vi "Verify Matching Board Capabilities.vi"(0 "TX Board Settings":T1[](array[typedef]) {"Address Space" items=["VXI/VME A16"=1, "VXI/VME A24"=2, "VXI/VME A32"=3, "VXI/VME A64"=4, "PXI Memory Allocations"=9, "PXI Configuration"=10, "PXI BAR0"=11, "PXI BAR1"=12, "PXI BAR2"=13, "PXI BAR3"=14, "PXI BAR4"=15, "PXI BAR5"=16]}, 1 "RX Board Settings":T1[](array[typedef]) {"Address Space" items=["VXI/VME A16"=1, "VXI/VME A24"=2, "VXI/VME A32"=3, "VXI/VME A64"=4, "PXI Memory Allocations"=9, "PXI Configuration"=10, "PXI BAR0"=11, "PXI BAR1"=12, "PXI BAR2"=13, "PXI BAR3"=14, "PXI BAR4"=15, "PXI BAR5"=16]}, 11 "error in (no error)":errorcluster) -> (4 "RX TX Board Settings":T1[](array[typedef]) {"Address Space" items=["VXI/VME A16"=1, "VXI/VME A24"=2, "VXI/VME A32"=3, "VXI/VME A64"=4, "PXI Memory Allocations"=9, "PXI Configuration"=10, "PXI BAR0"=11, "PXI BAR1"=12, "PXI BAR2"=13, "PXI BAR3"=14, "PXI BAR4"=15, "PXI BAR5"=16]}, 15 "error out":errorcluster)   [LabVIEW 2019]
uses:
  <instrlib>/niMmWave/ni3610 and ni3630/controls/public/Main Settings.ctl
  <vilib>/Instr/_visa.llb/VISA Register Access Address Space.ctl
  <instrlib>/niMmWave/ni3610 and ni3630/controls/public/Register Adresses.ctl
  <instrlib>/niMmWave/ni3610 and ni3630/controls/public/Base Card Type.ctl
  <instrlib>/niMmWave/ni3610 and ni3630/controls/private/IQ Card Revision.ctl
  <instrlib>/niMmWave/ni3610 and ni3630/controls/public/Board Capability.ctl
  <instrlib>/niMmWave/ni3610 and ni3630/ni3610_and_ni3630_Driver_Lib.lvlib
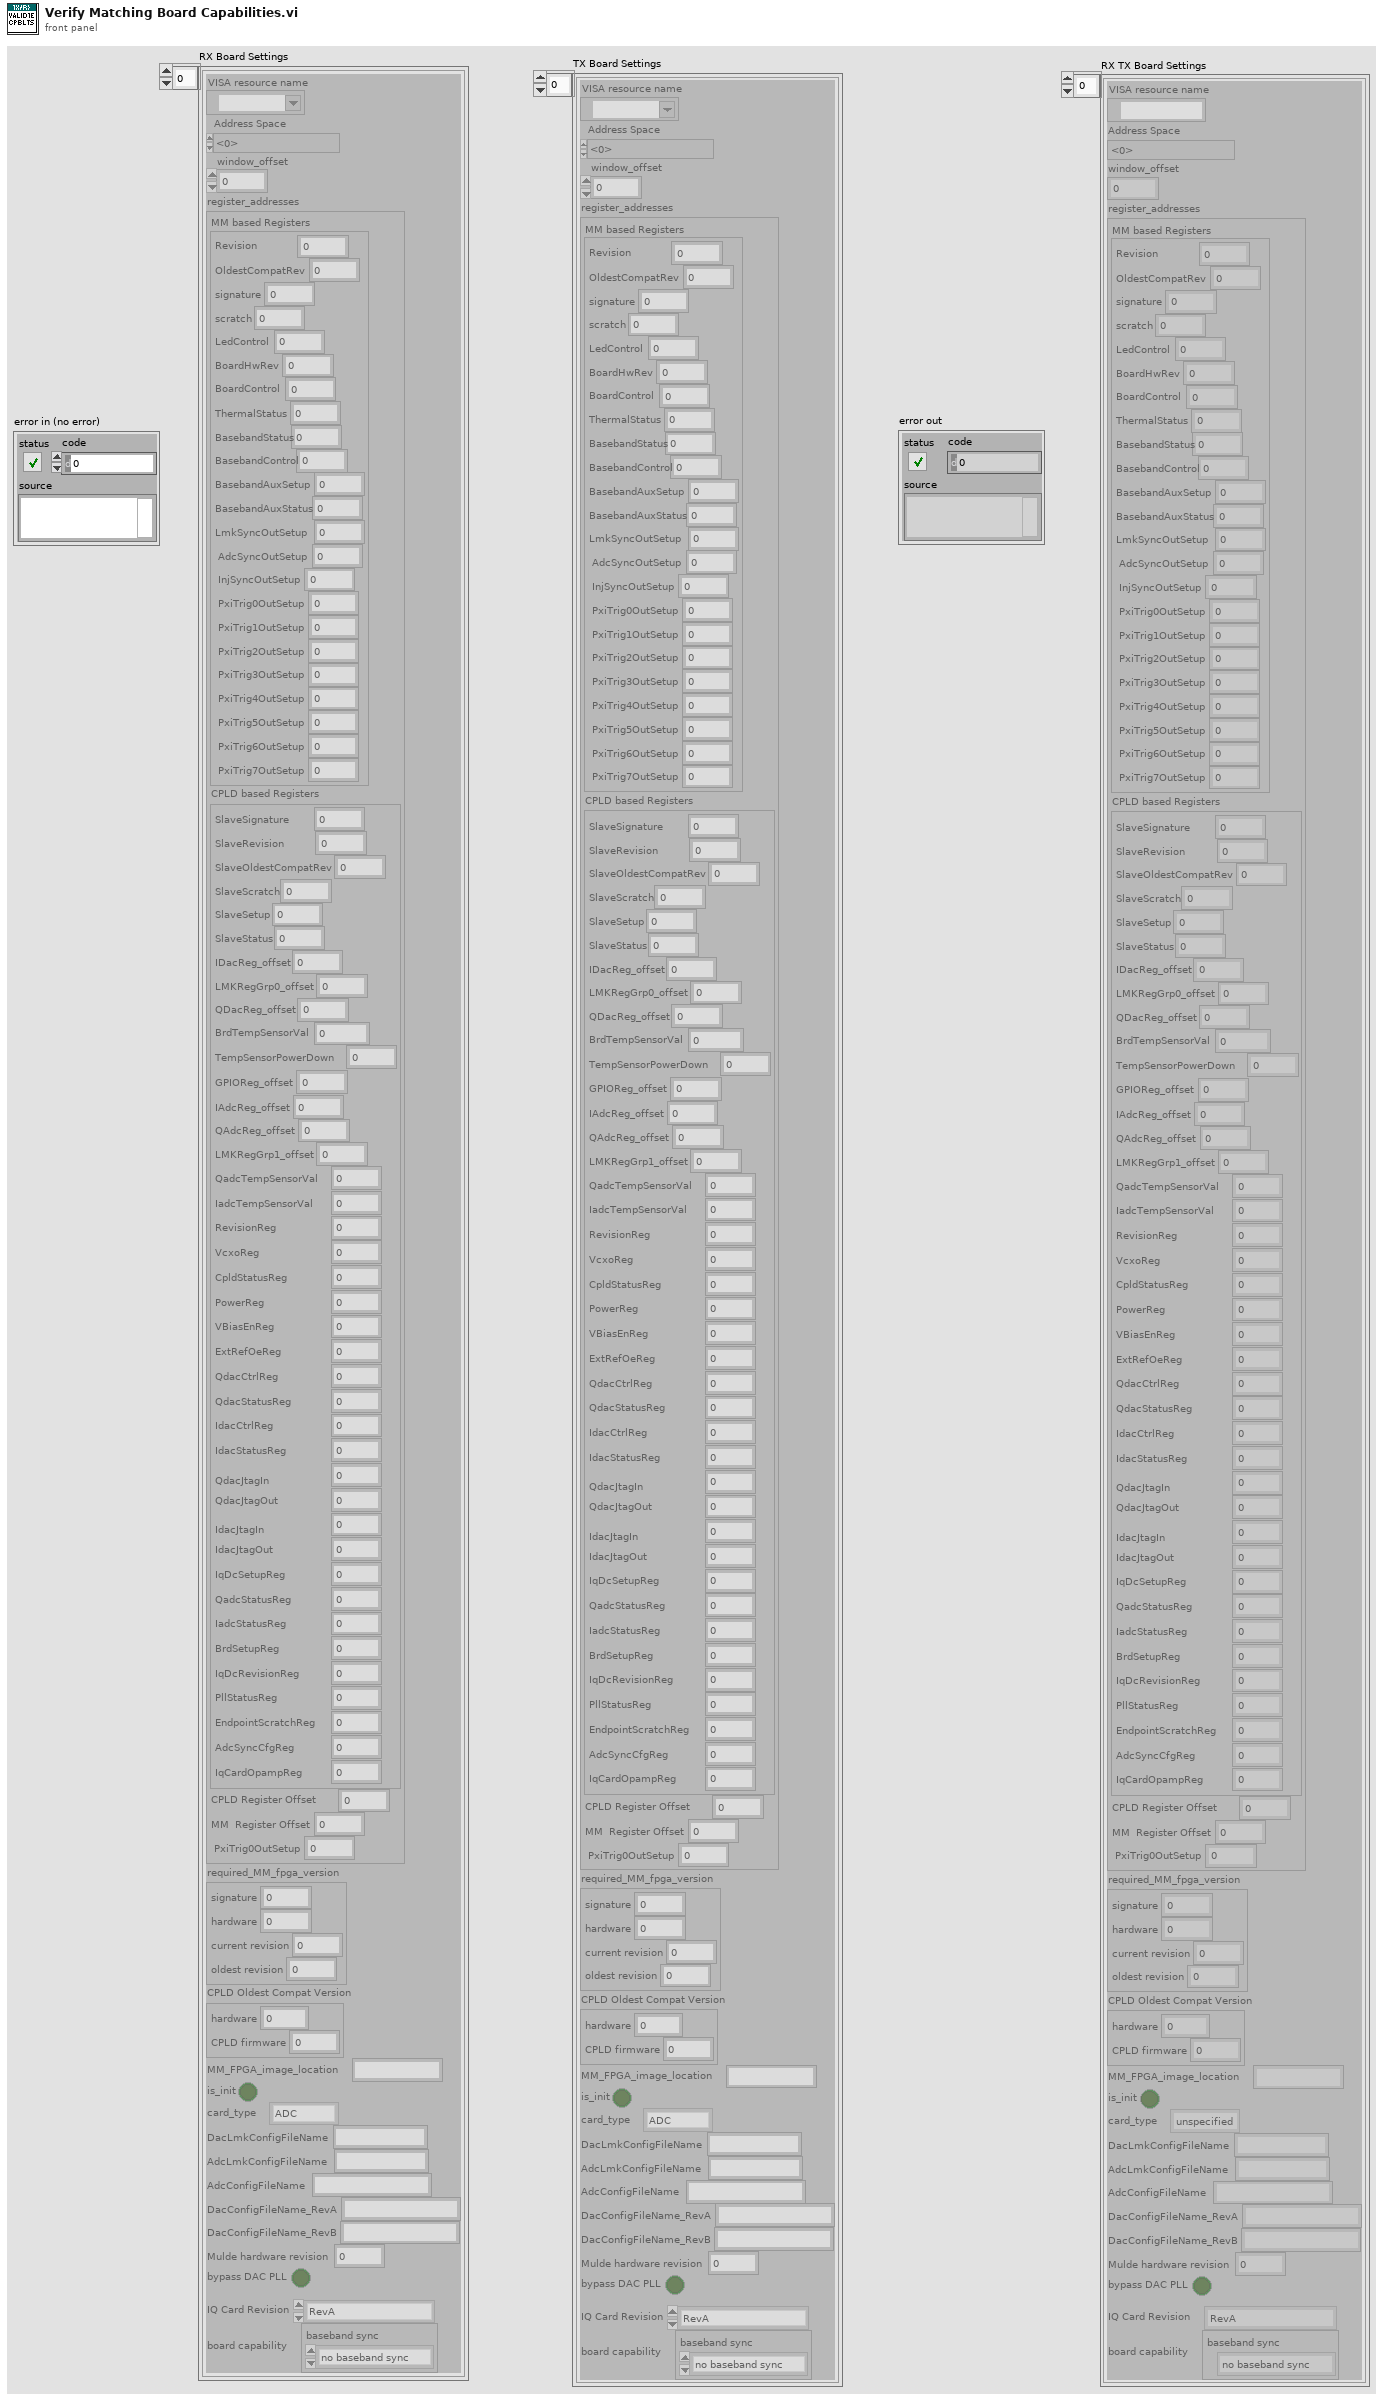
[diagram p1: front panel]
types:
  T1 = typedef "ni3610_and_ni3630_Driver_Lib.lvlib/Main Settings.ctl" = cluster{"VISA resource name":refnum<visa-resource-name>, "Address Space":T2, "window_offset":u32, "register_addresses":T3, "required_MM_fpga_version":cluster{"signature":u32, "hardware":u32, "current revision":u32, "oldest revision":u32}, "CPLD Oldest Compat Version ":cluster{"hardware":u32, "CPLD firmware":u32}, "MM_FPGA_image_location":string, "is_init":bool, "card_type":T4, "DacLmkConfigFileName":string, "AdcLmkConfigFileName":string, "AdcConfigFileName":string, "DacConfigFileName_RevA":string, "DacConfigFileName_RevB":string, "Mulde hardware revision":u8, "bypass DAC PLL\n":bool, "IQ Card Revision":T5, "board capability":T6}
  T2 = typedef "VISA Register Access Address Space.ctl" = u16
  T3 = typedef "ni3610_and_ni3630_Driver_Lib.lvlib/Register Adresses.ctl" = cluster{"MM based Registers":cluster{"Revision":u32, "OldestCompatRev":u32, "signature":u32, "scratch":u32, "LedControl":u32, "BoardHwRev":u32, "BoardControl":u32, "ThermalStatus":u32, "BasebandStatus":u32, "BasebandControl":u32, "BasebandAuxSetup":u32, "BasebandAuxStatus":u32, "LmkSyncOutSetup":u32, " AdcSyncOutSetup":u32, " InjSyncOutSetup":u32, " PxiTrig0OutSetup":u32, " PxiTrig1OutSetup":u32, " PxiTrig2OutSetup":u32, " PxiTrig3OutSetup":u32, " PxiTrig4OutSetup":u32, " PxiTrig5OutSetup":u32, " PxiTrig6OutSetup":u32, " PxiTrig7OutSetup":u32}, "CPLD based Registers":cluster{"SlaveSignature":u32, "SlaveRevision":u32, "SlaveOldestCompatRev":u32, "SlaveScratch":u32, "SlaveSetup":u32, "SlaveStatus":u32, "IDacReg_offset":u32, "LMKRegGrp0_offset":u32, "QDacReg_offset":u32, "BrdTempSensorVal":u32, "TempSensorPowerDown":u32, "GPIOReg_offset":u32, "IAdcReg_offset":u32, "QAdcReg_offset":u32, "LMKRegGrp1_offset":u32, "QadcTempSensorVal":u32, "IadcTempSensorVal":u32, "RevisionReg":u32, "VcxoReg":u32, "CpldStatusReg":u32, "PowerReg":u32, "VBiasEnReg":u32, "ExtRefOeReg":u32, "QdacCtrlReg":u32, "QdacStatusReg":u32, "IdacCtrlReg":u32, "IdacStatusReg":u32, "QdacJtagIn":u32, "QdacJtagOut":u32, "IdacJtagIn":u32, "IdacJtagOut":u32, "IqDcSetupReg":u32, "QadcStatusReg":u32, "IadcStatusReg":u32, "BrdSetupReg":u32, "IqDcRevisionReg":u32, "PllStatusReg":u32, "EndpointScratchReg":u32, "AdcSyncCfgReg":u32, "IqCardOpampReg":u32}, "CPLD Register Offset":u32, "MM  Register Offset":u32, " PxiTrig0OutSetup":u32}
  T4 = typedef "ni3610_and_ni3630_Driver_Lib.lvlib/Base Card Type.ctl" = enum16{"unspecified", "ADC", "DAC"}
  T5 = typedef "ni3610_and_ni3630_Driver_Lib.lvlib/IQ Card Revision.ctl" = enum16{"RevA", "RevB", "RevC", "RevD"}
  T6 = typedef "ni3610_and_ni3630_Driver_Lib.lvlib/Board Capability.ctl" = cluster{"baseband sync":enum16{"no baseband sync", "baseband sync"}}
  T7 = enum16{"no baseband sync", "baseband sync", "unknown hw"}
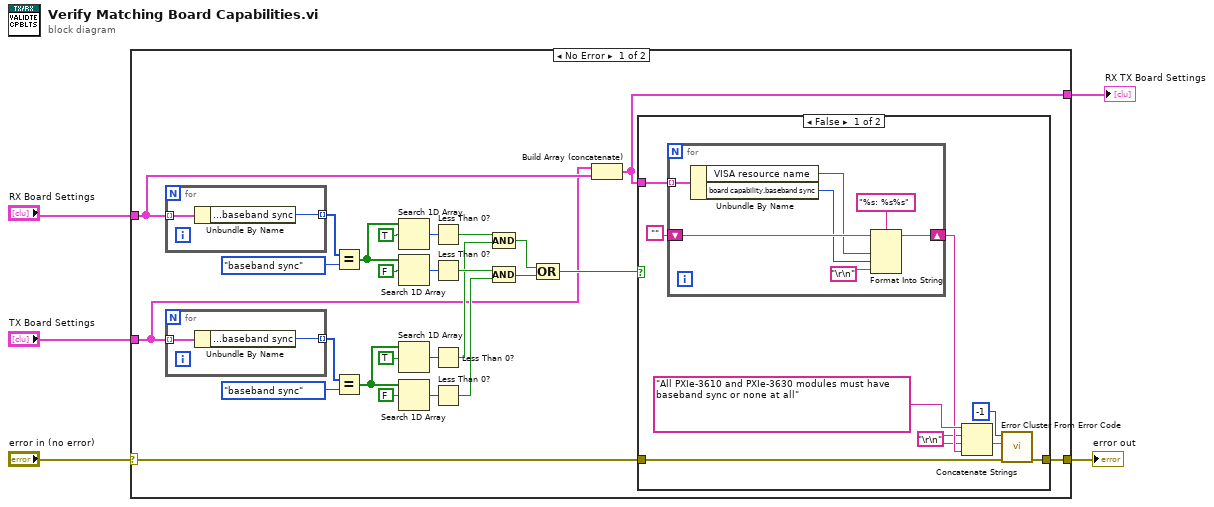
[diagram p0: block diagram]
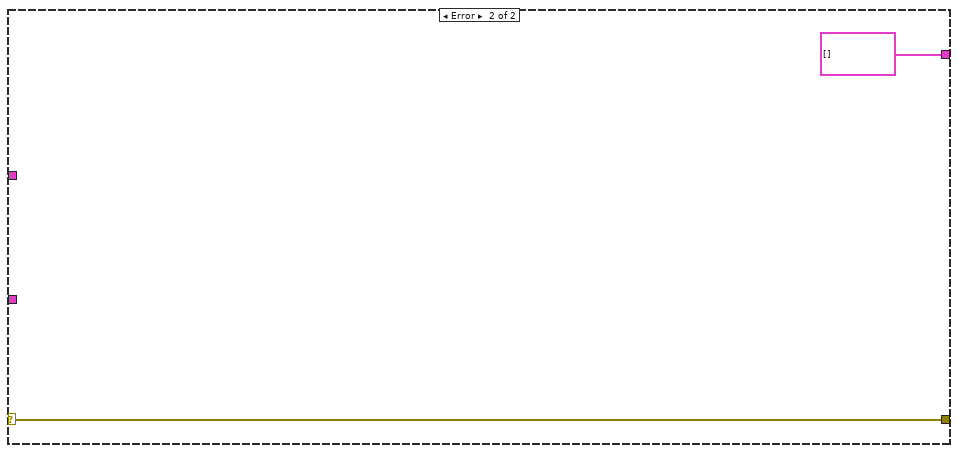
[diagram p3: hidden frame]
diagram:
  n1 = case shown="No Error" "error in (no error)" {
    selector: "error in (no error)" -> [w27 w54]
    tunnel: "TX Board Settings" -> [w7 _]
    tunnel: "RX Board Settings" -> [w8 _]
    tunnel: [w26 w54] -> w2
    tunnel: [w6 T1[] []] -> w1
    frame No Error {
      n2 = for {
        tunnel: w8 -> [w50] mode=indexing
        tunnel: [w49] -> w12 mode=indexing
        n3 = Unbundle By Name(w50) -> ("board capability.baseband sync"=w49:enum16{"no baseband sync", "baseband sync"})
      }
      n4 = for {
        tunnel: w7 -> [w52] mode=indexing
        tunnel: [w51] -> w11 mode=indexing
        n5 = Unbundle By Name(w52) -> ("board capability.baseband sync"=w51:enum16{"no baseband sync", "baseband sync"})
      }
      n6 = Equal?(x=w12, y=T7."baseband sync" ("board capability.baseband sync")) -> (x = y?=w21:bool[])
      n7 = Equal?(x=w11, y=T7."baseband sync" ("board capability.baseband sync")) -> (x = y?=w20:bool[])
      n8 = Search 1D Array(1D array=w21, element=TRUE) -> (index of element=w29:i32)  [unwired: 1 in]
      n9 = Search 1D Array(1D array=w21, element=FALSE) -> (index of element=w25:i32)  [unwired: 1 in]
      n10 = Search 1D Array(1D array=w20, element=TRUE) -> (index of element=w28:i32)  [unwired: 1 in]
      n11 = Search 1D Array(1D array=w20, element=FALSE) -> (index of element=w22:i32)  [unwired: 1 in]
      n12 = Less Than 0?(x=w29) -> (x < 0?=w19:bool)
      n13 = Less Than 0?(x=w25) -> (x < 0?=w18:bool)
      n14 = Less Than 0?(x=w28) -> (x < 0?=w17:bool)
      n15 = Less Than 0?(x=w22) -> (x < 0?=w16:bool)
      n16 = Compound Arithmetic op=AND(w19, w17) -> (w15:bool)
      n17 = Compound Arithmetic op=AND(w18, w16) -> (w14:bool)
      n18 = Compound Arithmetic op=OR(w15, w14) -> (w13:bool)
      n19 = Build Array (concatenate)(w7, w8) -> (w6:T1[])
      n20 = case shown="False" w13 {
        tunnel: w27 -> [w40 w48]
        tunnel: [w39 w48] -> w26
        tunnel: w6 -> [w37 _]
        frame False {
          w32 = "\r\n"
          n21 = for {
            tunnel: w37 -> [w46] mode=indexing
            shift-right: [w45] -> w33
            shift-left: "" -> [w44]
            n22 = Unbundle By Name(w46) -> ("VISA resource name"=w43:refnum<visa-resource-name>, "board capability.baseband sync"=w42:enum16{"no baseband sync", "baseband sync"})
            n23 = Format Into String(format string="%s: %s%s", initial string=w44, w43, w42, "\r\n") -> (resulting string=w45:string)  [unwired: 1 in, 1 out]
          }
          n24 = Concatenate Strings("All PXIe-3610 and PXIe-3630 modules must have baseband sync or none at all" ("error message (\"\")"), w32, w32, w33) -> (w36:string)
          n25 = call <vilib>:"Error Cluster From Error Code.vi"("error in (no error)"=w40, "error message (\"\")"=w36, "error code (0)"=-1) -> ("error out"=w39:errorcluster)  [unwired: 6 in]
        }
        frame True {
        }
      }
    }
    frame Error {
    }
  }
  "error out" <- w2
  "RX TX Board Settings" <- w1
